vi "Tomography.vi"() -> ()   [LabVIEW 2009]
uses:
  <vilib>/Analysis/Matrix/Datatypes/RealMatrix.ctl
  <vilib>/measure/matone.llb/Extract Single Tone Information 1 Chan.vi
  <vilib>/Analysis/3filter.llb/Butterworth Filter (DBL).vi
  <vilib>/Utility/file.llb/Read From Spreadsheet File (DBL).vi
  <vilib>/Analysis/7linalg.llb/Create Special Real Matrix.vi
  <vilib>/Analysis/NI_AALBase.lvlib
  <vilib>/measure/NI_MAPro.lvlib
  <vilib>/Analysis/NI_AALPro.lvlib
  <vilib>/Analysis/Matrix/NI_Matrix.lvlib
panel:
  in  "Number of Iterations":i32=100
  out "Rho":T1
  in  "Number of Photons":i32=10
  out "Regenerated phase wrapped 2":dbl[][](graph)
  out "detected phase (deg)":dbl format="%.2p"
  out "detected frequency":dbl format="%.4p"
  out "Regenerated phase wrapped":dbl[](graph)
  out "Normalized Envelope":waveform(dbl)(graph)
  out "Envelope":dbl[](graph)
  out "Normalized Squeezing":dbl[](graph)
  out "Normalized Noise":dbl[](graph)
  out "marginal size":i32
  out "Variances":dbl[](graph)
  out "sizeBin":dbl
  out "numpt":i32
  in  "Number of Bins":dbl=100.0
  in  "Shot":path=path "F:/data/tomo final/shotfinal.txt"
  in  "Squeezing":path=path "F:/data/tomo final/sqzfinal.txt"
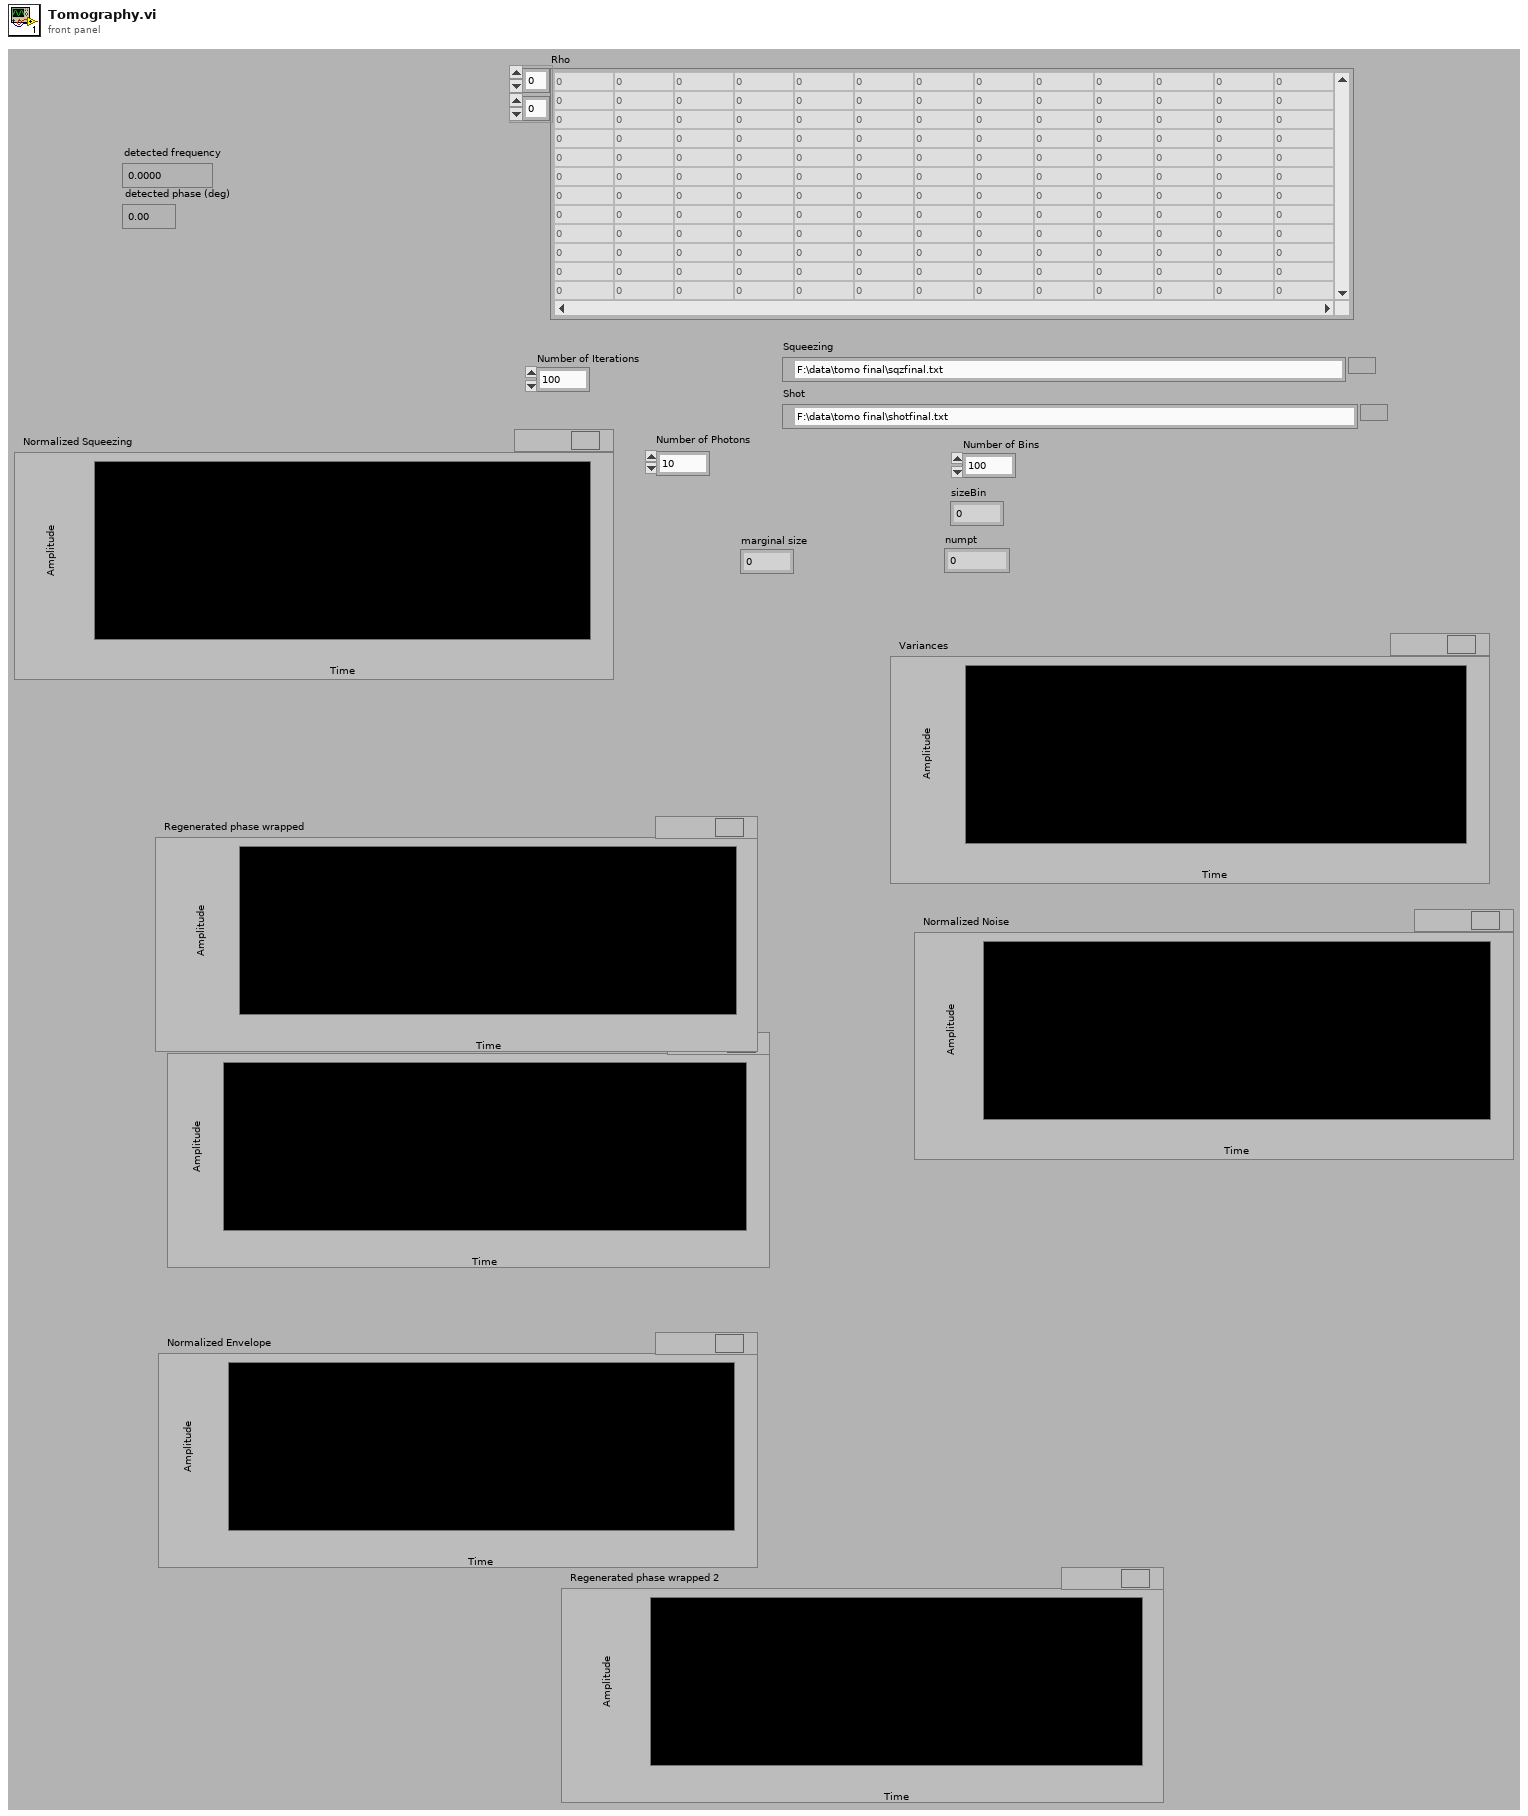
[diagram p1: front panel]
types:
  T1 = typedef "NI_Matrix.lvlib/RealMatrix.ctl" = dbl[][]
  T2 = enum32{"Identity", "Diagonal", "Toepliz", "Vandermonde", "Companion"}
  T3 = enum32{"Lowpass", "Highpass", "Bandpass", "Bandstop"}
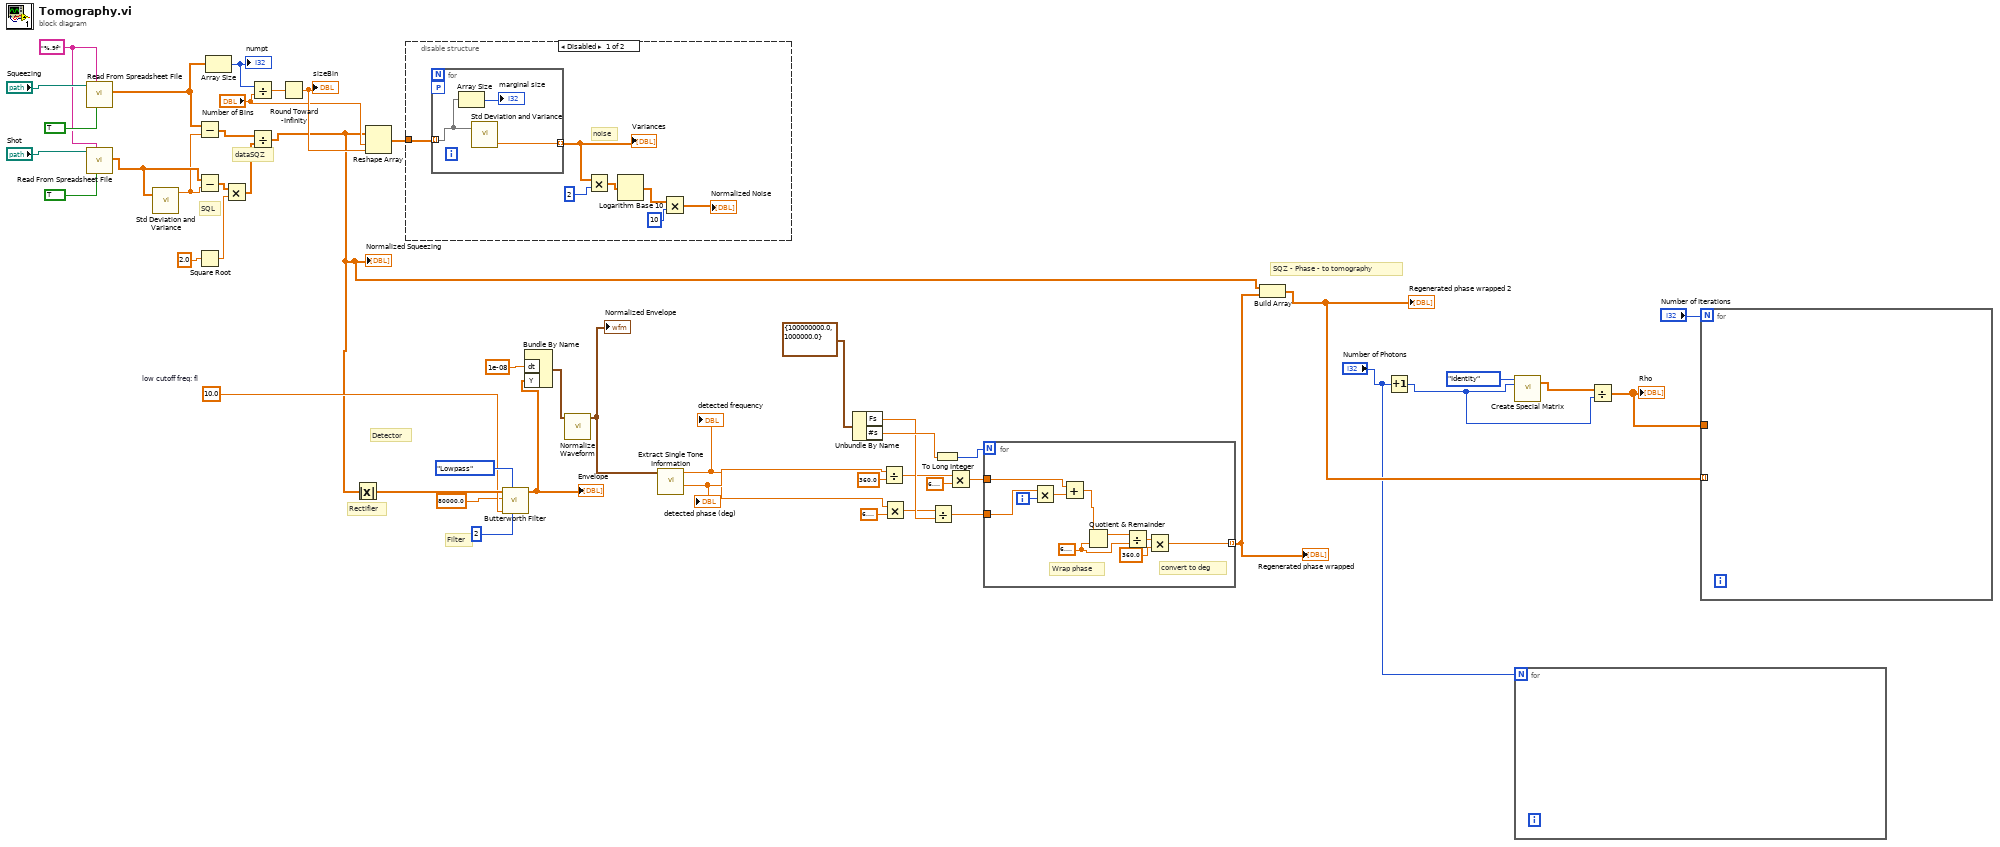
[diagram p0: block diagram]
diagram:
  w29 = 10.0  # low cutoff freq: fl
  w47 = "%.9f" ("format (%.3f)")
  # "SQZ - Phase - to tomography"
  # "Detector"
  # "Filter"
  # "Rectifier"
  # "dataSQZ"
  # "SQL"
  n1 = call-poly <vilib>:"Read From Spreadsheet File.vi"("transpose (no:F)"=TRUE, "format (%.3f)"=w47, "file path (dialog if empty)"="Squeezing") -> ("first row"=w37:dbl[])  [unwired: 4 in, 4 out]
  n2 = call-poly <vilib>:"Read From Spreadsheet File.vi"("transpose (no:F)"=TRUE, "format (%.3f)"=w47, "file path (dialog if empty)"="Shot") -> ("first row"=w44:dbl[])  [unwired: 4 in, 4 out]
  n3 = call <vilib>:"Std Deviation and Variance.vi"("X"=w44) -> ("mean"=w43:dbl)  [unwired: 1 in, 2 out]
  n4 = Subtract(x=w37, y=w43) -> (x-y=w42:dbl[])
  n5 = Subtract(x=w44, y=w43) -> (x-y=w39:dbl[])
  n6 = Square Root(x=2.0) -> (sqrt(x)=w40:dbl)
  n7 = Array Size(array=w37) -> (size(s)=w36:i32)
  "numpt" <- w36
  n8 = Multiply(x=w39, y=w40) -> (x*y=w38:dbl[])
  n9 = Divide(x=w36, y="Number of Bins") -> (x/y=w35:dbl)
  n10 = Divide(x=w42, y=w38) -> (x/y=w8:dbl[])
  "Normalized Squeezing" <- w8
  n11 = Round Toward -Infinity(1:w35) -> (0:w33:dbl)
  "sizeBin" <- w33
  n12 = Absolute Value(x=w8) -> (abs(x)=w30:dbl[])
  n13 = Reshape Array(w8, "Number of Bins", w33) -> (w34:dbl[][])
  n14 = disable-structure shown="Disabled" {
    disable-tunnel: w34 -> [w56 _]
    frame #0 {
      # "noise"
      n15 = for {
        tunnel: w56 -> [w58] mode=indexing
        tunnel: [w59] -> w54 mode=indexing
        workers-P: _ -> [_]
        n16 = Array Size(array=w58) -> (size(s)=→"marginal size":i32)
        n17 = call <vilib>:"Std Deviation and Variance.vi"("X"=w58) -> ("variance"=w59:dbl)  [unwired: 1 in, 2 out]
      }
      "Variances" <- w54
      n18 = Multiply(x=w54, y=2) -> (x*y=w55:dbl[])
      n19 = Logarithm Base 10(1:w55) -> (0:w52:dbl[])
      n20 = Multiply(x=w52, y=10) -> (x*y=→"Normalized Noise":dbl[])
    }
    frame #1 {
    }
  }
  n21 = call-poly <vilib>:"Butterworth Filter.vi"("order"=2, "filter type"=T3."Lowpass", "low cutoff freq: fl"=w29, "sampling freq: fs"=80000.0, "X"=w30) -> ("Filtered X"=w10:dbl[])  [unwired: 3 in, 1 out]
  "Envelope" <- w10
  n22 = Bundle By Name("dt"=1e-08, "Y"=w10) -> (w25:waveform(dbl))  [unwired: 1 in]
  n23 = call <vilib>:"Normalize Waveform.vi"("waveform in"=w25) -> ("normalized waveform"=w24:waveform(dbl))  [unwired: 7 in, 3 out]
  "Normalized Envelope" <- w24
  n24 = call-poly <vilib>:"Extract Single Tone Information.vi"("time signal in"=w24) -> ("detected phase (deg)"=w12:dbl, "detected frequency"=w11:dbl)  [unwired: 5 in, 4 out]
  "detected frequency" <- w11
  "detected phase (deg)" <- w12
  n25 = Unbundle By Name(cluster{"Fs":dbl, "#s":dbl} {"Fs"=100000000.0, "#s"=1000000.0} ("sampling info")) -> ("Fs"=w21:dbl, "#s"=w22:dbl)
  n26 = Divide(x=w12, y=360.0) -> (x/y=w15:dbl)
  n27 = Multiply(x=w11, y=6.283185307179586) -> (x*y=w18:dbl)
  n28 = Divide(x=w18, y=w21) -> (x/y=w19:dbl)
  n29 = To Long Integer(number=w22) -> (32bit integer=w23:i32)
  n30 = Multiply(x=w15, y=6.283185307179586) -> (x*y=w20:dbl)
  n31 = for {
    N: w23 -> [_]
    tunnel: w19 -> [w68]
    tunnel: w20 -> [w67]
    tunnel: [w62] -> w9 mode=indexing
    i -> [w69]
    w65 = 6.283185307179586
    # "convert to deg"
    # "Wrap phase"
    n32 = Multiply(x=w68, y=w69) -> (x*y=w66:dbl)
    n33 = Add(x=w67, y=w66) -> (x+y=w61:dbl)
    n34 = Quotient & Remainder(x=w61, y=w65) -> (x-y*floor(x/y)=w60:dbl)  [unwired: 1 out]
    n35 = Divide(x=w60, y=w65) -> (x/y=w64:dbl)
    n36 = Multiply(x=w64, y=360.0) -> (x*y=w62:dbl)
  }
  "Regenerated phase wrapped" <- w9
  n37 = Build Array(w8, w9) -> (w2:dbl[][])
  "Regenerated phase wrapped 2" <- w2
  n38 = Increment(x="Number of Photons") -> (x+1=w5:i32)
  n39 = call-poly <vilib>:"Create Special Matrix.vi"("matrix type"=T2."Identity", "matrix size"=w5) -> ("Special Matrix"=w6:T1)  [unwired: 3 in, 1 out]
  n40 = for {
    N: "Number of Photons" -> [_]
  }
  n41 = Divide(x=w6, y=w5) -> (x/y=w3:T1)
  "Rho" <- w3
  n42 = for {
    N: "Number of Iterations" -> [_]
    tunnel: w3 -> [_]
    tunnel: w2 -> [_] mode=indexing
  }
